vi "Run All.vi"(8 "error in (no error)":errorcluster, 11 "Thread Manager in":refnum<class "Thread Manager.lvclass">) -> (0 "error out":errorcluster, 3 "Thread Manager out":refnum<class "Thread Manager.lvclass">)   [LabVIEW 2017, in "DSF Core.lvlib" / "Thread Manager.lvclass"]
uses:
  Thread Manager.lvclass
  Thread Manager.lvclass/Thread Manager.ctl
  Thread/Thread.lvclass
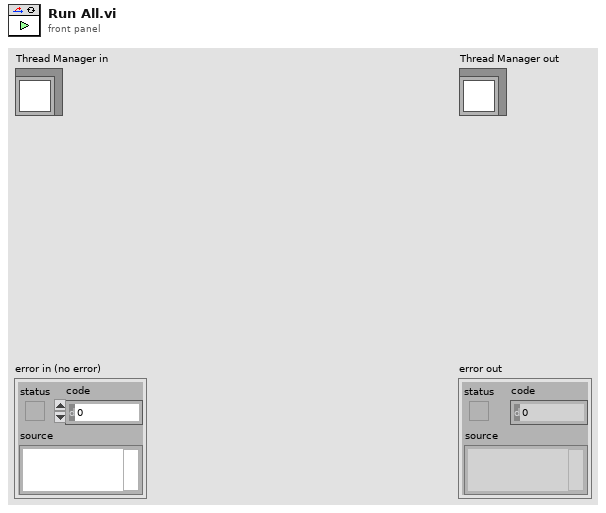
[diagram p1: front panel]
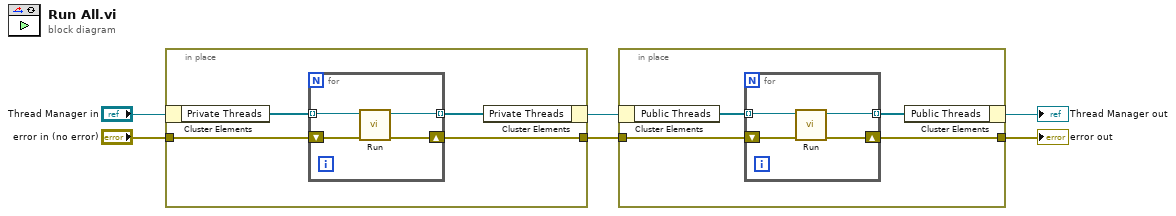
[diagram p0: block diagram]
diagram:
  n1 = in-place {
    in-place-border: [w8] -> w3
    in-place-border: "error in (no error)" -> [w7]
    n2 = in-place-cluster #1("Thread Manager in") -> ("Private Threads"=w10:refnum<class "Thread.lvclass">[])
    n3 = for {
      tunnel: w10 -> [w14] mode=indexing
      tunnel: [w13] -> w9 mode=indexing
      shift-right: [w12] -> w8
      shift-left: w7 -> [w11]
      n4 = call "Run.vi"("error in (no error)"=w11, "Thread in"=w14) -> ("error out"=w12:errorcluster, "Thread out"=w13:refnum<class "Thread.lvclass">)  [unwired: 8 in]
    }
    n5 = in-place-cluster #1("Private Threads"=w9) -> (w4:refnum<class "Thread Manager.lvclass">)
  }
  n6 = in-place {
    in-place-border: [w16] -> w2
    in-place-border: w3 -> [w15]
    n7 = in-place-cluster #2(w4) -> ("Public Threads"=w18:refnum<class "Thread.lvclass">[])
    n8 = for {
      tunnel: w18 -> [w22] mode=indexing
      tunnel: [w21] -> w17 mode=indexing
      shift-right: [w20] -> w16
      shift-left: w15 -> [w19]
      n9 = call "Run.vi"("error in (no error)"=w19, "Thread in"=w22) -> ("error out"=w20:errorcluster, "Thread out"=w21:refnum<class "Thread.lvclass">)  [unwired: 8 in]
    }
    n10 = in-place-cluster #2("Public Threads"=w17) -> (→"Thread Manager out":refnum<class "Thread Manager.lvclass">)
  }
  "error out" <- w2
